vi "Write generation type.vi"(8 "error in (no error)":errorcluster, 10 "generation type":T1, 11 "AudioGeneration in":refnum<class "AudioGeneration.lvclass">) -> (0 "error out":errorcluster, 3 "AudioGeneration out":refnum<class "AudioGeneration.lvclass">)   [LabVIEW 2021, in "AudioGeneration.lvclass"]
uses:
  AudioGeneration.lvclass
  AudioGeneration.lvclass/AudioGeneration.ctl
  controls/generation type.ctl
  controls/AudioGenTypeDefs.lvlib
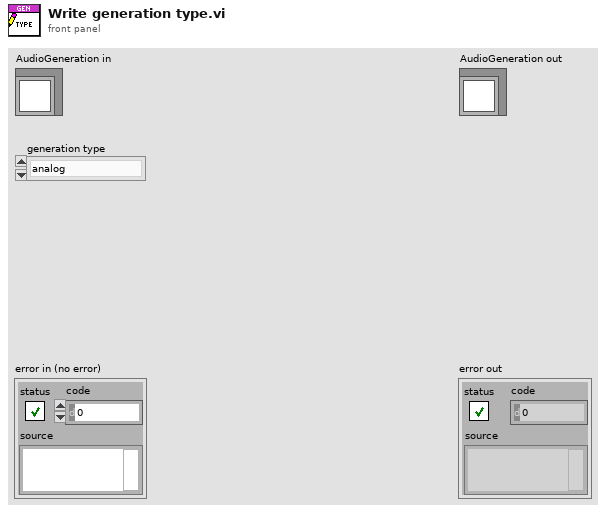
[diagram p1: front panel]
types:
  T1 = typedef "AudioGenTypeDefs.lvlib/generation type.ctl" = enum16{"analog", "digital"}
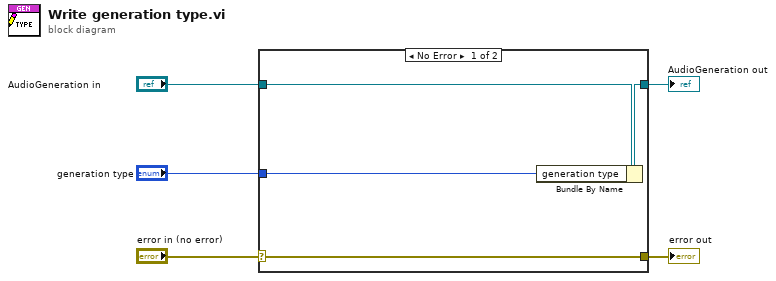
[diagram p0: block diagram]
diagram:
  n1 = case shown="No Error" "error in (no error)" {
    selector: "error in (no error)" -> [w9 w10]
    tunnel: [w9 w10] -> w4
    tunnel: [w7 w11] -> w2
    tunnel: "AudioGeneration in" -> [w8 w11]
    tunnel: "generation type" -> [w6 _]
    frame No Error {
      n2 = Bundle By Name(cluster=w8, "generation type"=w6) -> (w7:refnum<class "AudioGeneration.lvclass">)
    }
    frame Error {
    }
  }
  "error out" <- w4
  "AudioGeneration out" <- w2
